vi "Sort data for upload.vi"(7 "Add reset (T)":bool=TRUE, 9 "Colour array in":u32[](array[numeric]), 10 "Zero Outputs?":bool, 11 "ID":u32) -> (3 "Upload data":u32[](array[numeric]))   [LabVIEW 2015]
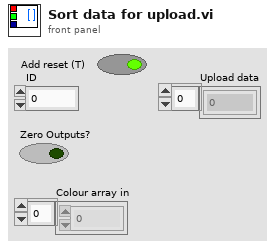
[diagram p1: front panel]
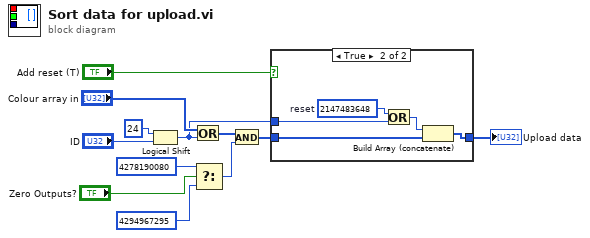
[diagram p0: block diagram]
diagram:
  n1 = Logical Shift(y=i16 24, x="ID") -> (x << y=w1:u32)
  n2 = Or(x="Colour array in", y=w1) -> (x .or. y?=w12:u32[])
  n3 = Select(t=u32 4278190080, s="Zero Outputs?", f=u32 4294967295) -> (s? t:f=w7:u32)
  n4 = And(x=w12, y=w7) -> (x .and. y?=w6:u32[])
  n5 = case shown="True" "Add reset (T)" {
    tunnel: w6 -> [w13 w18]
    tunnel: [w13 w17] -> w5
    tunnel: w1 -> [_ w15]
    frame False {
    }
    frame True {
      w14 = u32 2147483648  # reset
      n6 = Or(x=w14, y=w15) -> (x .or. y?=w16:u32)
      n7 = Build Array (concatenate)(w16, w18) -> (w17:u32[])
    }
  }
  "Upload data" <- w5
